vi "Read Auto Load.vi"(8 "error in (no error)":errorcluster, 11 "ProjectLoader in":refnum<class "ProjectLoader.lvclass">) -> (0 "error out":errorcluster, 2 "Auto Load":bool, 3 "ProjectLoader out":refnum<class "ProjectLoader.lvclass">)   [LabVIEW 2015, in "ProjectLoader.lvclass"]
uses:
  ProjectLoader.lvclass
  ProjectLoader.lvclass/ProjectLoader.ctl
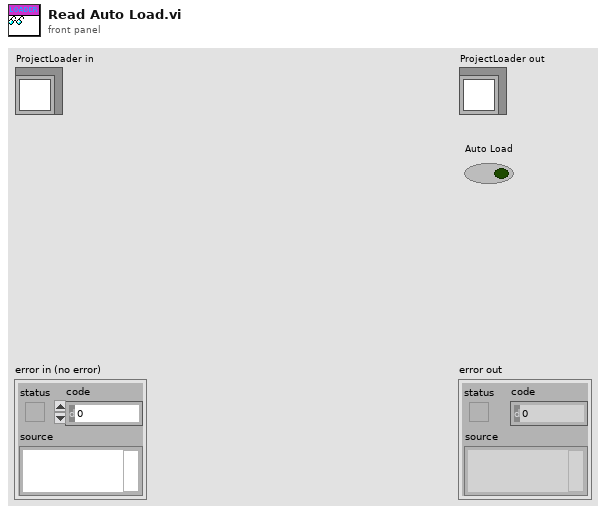
[diagram p1: front panel]
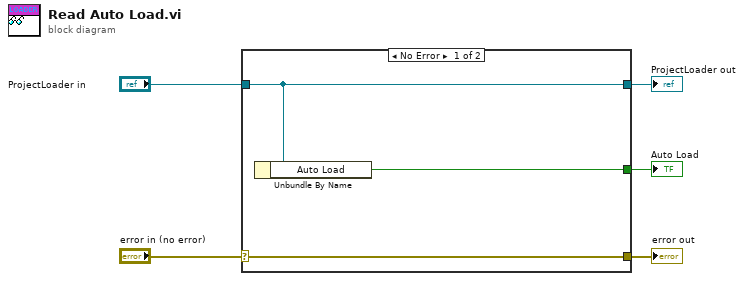
[diagram p0: block diagram]
diagram:
  n1 = case shown="No Error" "error in (no error)" {
    selector: "error in (no error)" -> [w8 w9]
    tunnel: [w8 w9] -> w4
    tunnel: [w7 w10] -> w2
    tunnel: "ProjectLoader in" -> [w7 w10]
    tunnel: [w6 _] -> w1
    frame No Error {
      n2 = Unbundle By Name(w7) -> ("Auto Load"=w6:bool)
    }
    frame Error {
    }
  }
  "error out" <- w4
  "ProjectLoader out" <- w2
  "Auto Load" <- w1
